vi "Q1_Al_Arthur.vi"() -> ()   [LabVIEW 2019]
uses:
  <vilib>/Utility/file.llb/Read Delimited Spreadsheet (DBL).vi
panel:
  out "Waveform Chart 2":dbl[][](graph)
  out "Waveform Chart":dbl[][](graph)
  in  "file path  2":path
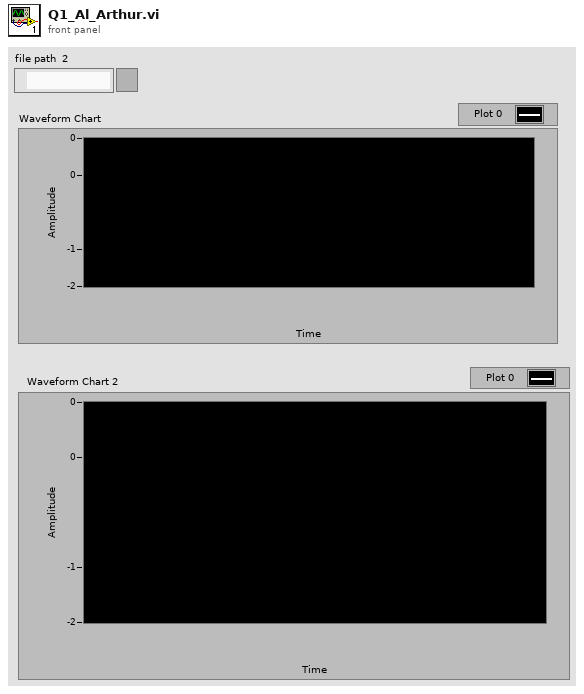
[diagram p1: front panel]
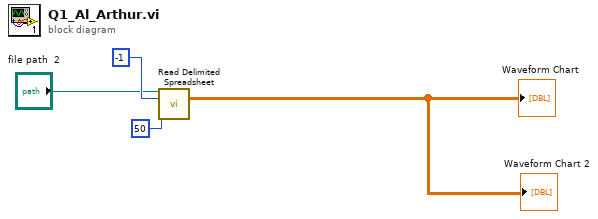
[diagram p0: block diagram]
diagram:
  n1 = call-poly <vilib>:"Read Delimited Spreadsheet.vi"("file path (dialog if empty)"="file path  2", "number of rows (all:-1)"=-1, "max characters/row  (no limit:0)"=50) -> ("all rows"=→"Waveform Chart" →"Waveform Chart 2":dbl[][])  [unwired: 7 in, 5 out]
